vi "Data Length.vi"(1 "Data Length U8 []":u8[](array[numeric])) -> (0 "Data Length":u32)   [LabVIEW 2020, in "SECS Communication.lvlib" / "SECS-II Class.lvclass"]
uses:
  SECS-II Class.lvclass
  SECS-II Class.lvclass/SECS-II Class.ctl
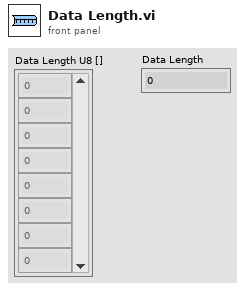
[diagram p1: front panel]
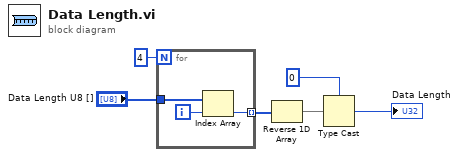
[diagram p0: block diagram]
diagram:
  n1 = for {
    N: 4 -> [_]
    tunnel: "Data Length U8 []" -> [w9]
    tunnel: [w7] -> w4 mode=indexing
    i -> [w8]
    n2 = Index Array(array=w9, index=w8) -> (element=w7:u8)
  }
  n3 = Reverse 1D Array(array=w4) -> (reversed array=w3:u8[])
  n4 = Type Cast(type=u32 0, x=w3) -> (*(type *) &x=→"Data Length":u32)
